vi "convertVecToArray.vi"(1 "Channels":i32, 2 "buffer in":dbl[](array[numeric])) -> (0 "Array":dbl[][](array[numeric]))   [LabVIEW 2024]
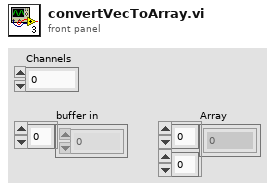
[diagram p1: front panel]
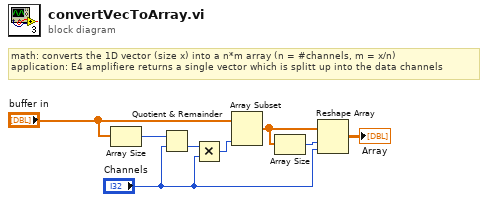
[diagram p0: block diagram]
diagram:
  # "math: converts the 1D vector (size x) into a n*m array (n = #channels, m = x/n)\napplication: E4 amplifiere returns a single vector which is splitt up into the data channels"
  n1 = Array Size(array="buffer in") -> (size(s)=w3:i32)
  n2 = Quotient & Remainder(x=w3, y="Channels") -> (floor(x/y)=w5:i32)  [unwired: 1 out]
  n3 = Multiply(x=w5, y="Channels") -> (x*y=w4:i32)
  n4 = Array Subset(array="buffer in", length=w4) -> (w6:dbl[])  [unwired: 1 in]
  n5 = Array Size(array=w6) -> (size(s)=w7:i32)
  n6 = Reshape Array(w6, w7, "Channels") -> (→"Array":dbl[][])
